vi "Override Error.vi"(10 "Error":errorcluster={"status"=FALSE, "code"=0, "source"="e3b0c44298fc1c149afbf4c8996fb92427ae41e4649b934ca495991b7852b855"}, 11 "jettl Queue Actor in":refnum<class "jettl Queue Actor.lvclass">) -> (3 "jettl Queue Actor out":refnum<class "jettl Queue Actor.lvclass">)   [LabVIEW 2021, in "jettl.lvlib" / "jettl Queue Actor.lvlib" / "jettl Queue Actor.lvclass"]
uses:
  jettl Queue Actor.lvclass
  <vilib>/Utility/error.llb/DialogType.ctl
  jettl Queue Actor.lvclass/jettl Queue Actor.ctl
panel:
  # "source default set to SHA256."
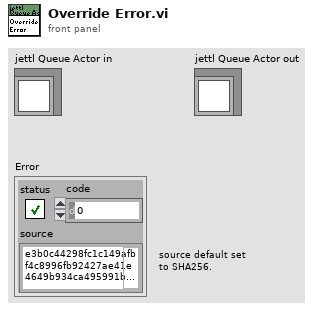
[diagram p1: front panel]
types:
  T1 = typedef "DialogType.ctl" = u16
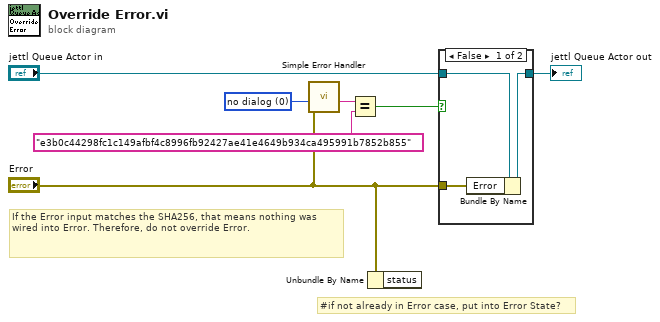
[diagram p0: block diagram]
diagram:
  w4 = T1 0 items=["no dialog", "OK message", "continue or stop message", "OK message + warnings", "continue/stop + warnings"] ("type of dialog (OK msg:1)")
  # "#if not already in Error case, put into Error State?"
  # "If the Error input matches the SHA256, that means nothing was wired into Error. Therefore, do not override Error."
  n1 = call <vilib>:"Simple Error Handler.vi"("type of dialog (OK msg:1)"=w4, "error in (no error)"="Error") -> ("source out"=w3:string)  [unwired: 3 in, 4 out]
  n2 = Equal?(x=w3, y="e3b0c44298fc1c149afbf4c8996fb92427ae41e4649b934ca495991b7852b855") -> (x = y?=w2:bool)
  n3 = Unbundle By Name("Error") -> ()  [unwired: 1 out]
  n4 = case shown="False" w2 {
    tunnel: "jettl Queue Actor in" -> [w10 w11]
    tunnel: [w9 w11] -> w6
    tunnel: "Error" -> [w8 _]
    frame False {
      n5 = Bundle By Name(cluster=w10, "Error"=w8) -> (w9:refnum<class "jettl Queue Actor.lvclass">)
    }
    frame True {
    }
  }
  "jettl Queue Actor out" <- w6
